vi "Core_Module.vi"(11 "Error_In":errorcluster) -> (4 "Obtained_PSRR_Data":T1, 6 "Last_Read_PSRR (dB)":i32, 8 "Last_Error_Details":T4 caption="Last Error Details", 14 "Colors [4]":T3={"Error?_Color"=[], "Error?_Text"="No_Error"}, 15 "Error_Out":errorcluster)   [LabVIEW 2021]
doc: "Core module perform most of the execution of the application."
uses:
  <vilib>/regexp/Match Regular Expression.xnode
  Controls/Last_Error_Details.ctl
  Controls/BI_Error_Con.ctl
  Controls/Obtained_PSRR_Data.ctl
  Controls/Obtained_PSRR_Data_Operation.ctl
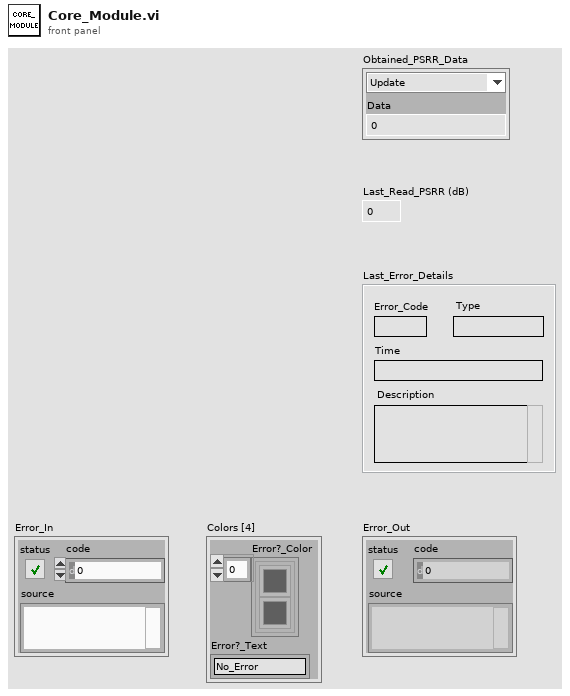
[diagram p1: front panel]
types:
  T1 = typedef "Obtained_PSRR_Data.ctl" = cluster{"Data":i32, "Obtained_PSRR_Data_Operation":T2}
  T2 = typedef "Obtained_PSRR_Data_Operation.ctl" = enum16{"Update", "Dont_Update", "Clear"}
  T3 = typedef "BI_Error_Con.ctl" = cluster{"Error?_Color":cluster{u32, u32}[], "Error?_Text":string}
  T4 = typedef "Last_Error_Details.ctl" = cluster{"Error_Code":string, "Type":string, "Time":string, "Description":string}
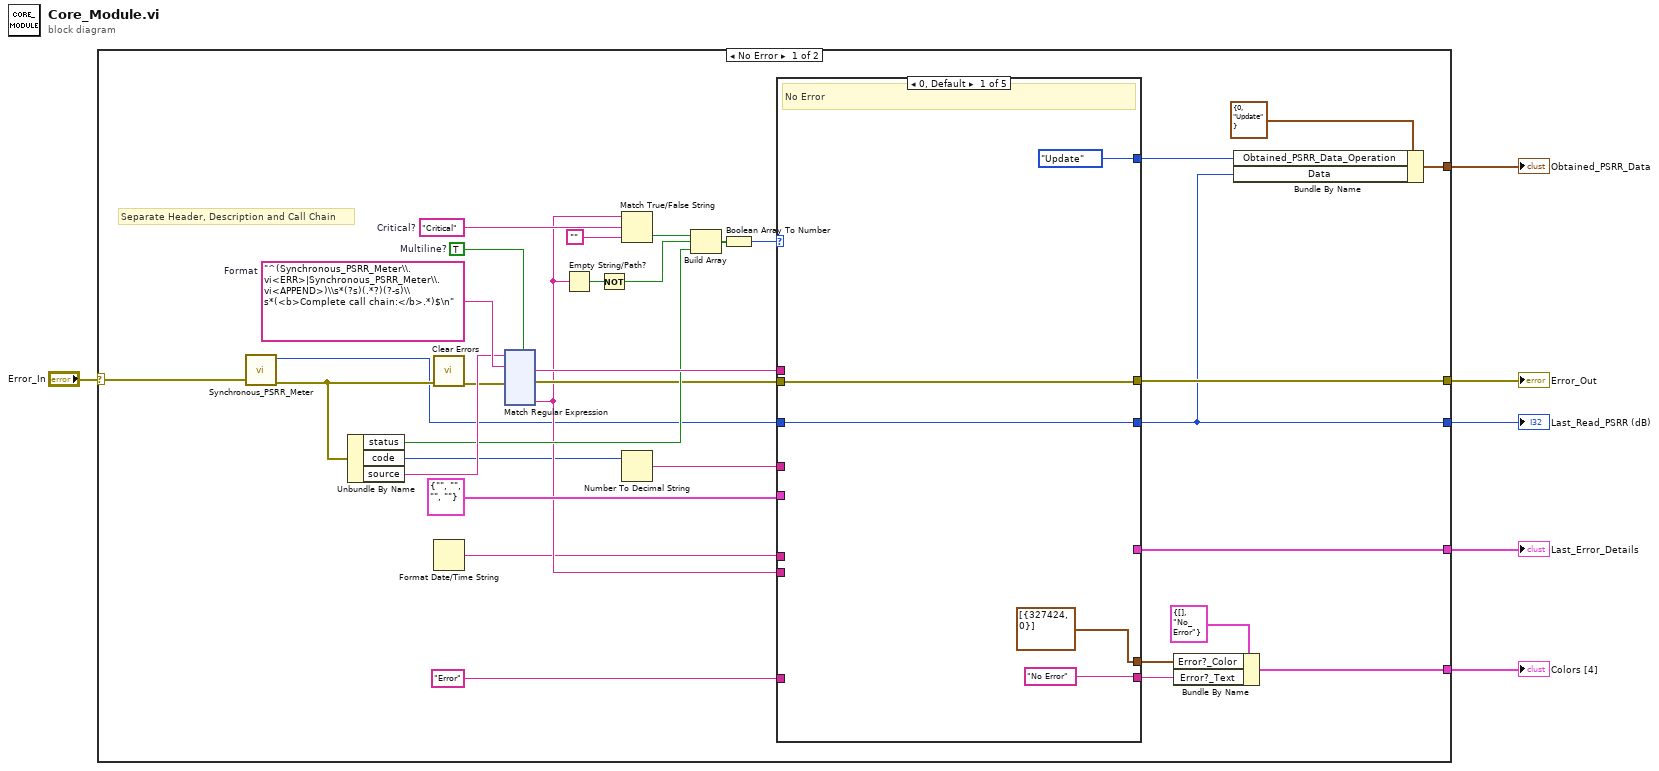
[diagram p0: block diagram]
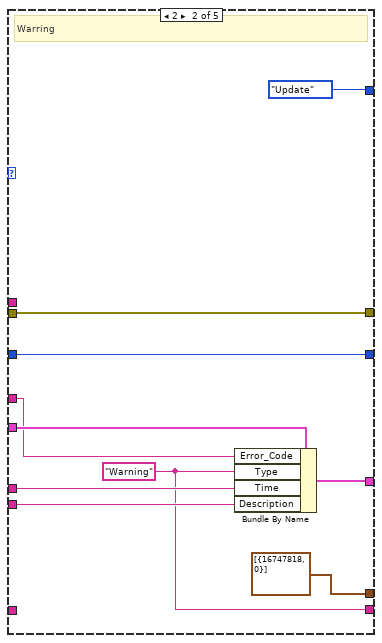
[diagram p2: hidden frame]
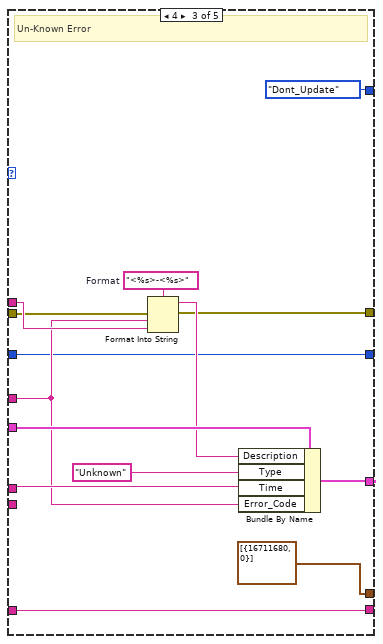
[diagram p3: hidden frame]
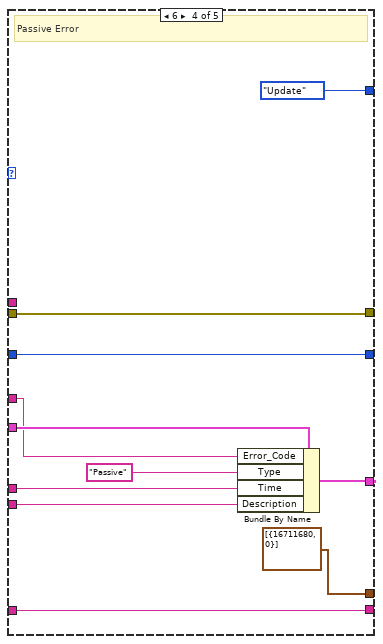
[diagram p4: hidden frame]
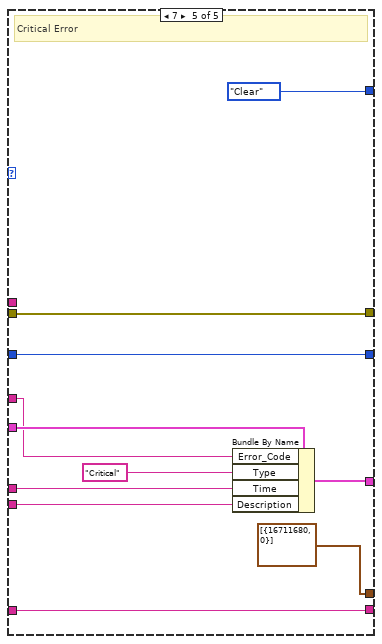
[diagram p5: hidden frame]
diagram:
  n1 = case shown="No Error" "Error_In" {
    selector: "Error_In" -> [w7 w211]
    tunnel: [w26 w211] -> w2
    tunnel: [w12 _] -> w5
    tunnel: [w15 _] -> w6
    tunnel: [w14 _] -> w4
    tunnel: [w19 _] -> w3
    frame No Error {
      w36 = "Critical"  # Critical?
      w38 = TRUE  # Multiline?
      w39 = "^(Synchronous_PSRR_Meter\\.vi<ERR>|Synchronous_PSRR_Meter\\.vi<APPEND>)\\s*(?s)(.*?)(?-s)\\s*(<b>Complete call chain:</b>.*)$\n"  # Format
      # "Separate Header, Description and Call Chain"
      n2 = call "Synchronous_PSRR_Meter.vi"("error in"=w7) -> ("error out"=w9:errorcluster, "PSRR (dB)"=w8:i32)  [unwired: 9 in]
      n3 = Unbundle By Name(w9) -> ("status"=w29:bool, "code"=w22:i32, "source"=w33:string)
      n4 = call <vilib>:"Clear Errors.vi"("error in (no error)"=w9) -> ("error out"=w20:errorcluster)  [unwired: 5 in, 1 out]
      n5 = Format Date/Time String() -> (date/time string=w10:string)  [unwired: 3 in]
      n6 = xnode "Match Regular Expression"("input string"=w33, "regular expression"=w39, "error in"=w20, "multiline? (F)"=w38) -> ("after match"=w37:string, "error out"=w25:errorcluster, "submatch 2"=w24:string)  [unwired: 2 in, 4 out]
      n7 = Empty String/Path?(string/path=w24) -> (empty?=w34:bool)
      n8 = Not(x=w34) -> (.not. x?=w27:bool)
      n9 = Match True/False String(2:"" ("false string"), 3:w36, 4:w24) -> (0:w28:bool)  [unwired: 1 out]
      n10 = Number To Decimal String(number=w22) -> (decimal integer string=w21:string)  [unwired: 1 in]
      n11 = Build Array(w28, w27, w29) -> (w32:bool[])
      n12 = Boolean Array To Number(Boolean array=w32) -> (number=w31:u32)
      n13 = case shown="0, Default" w31 {
        tunnel: w8 -> [w164 w170 w180 w190 w207]
        tunnel: w24 -> [_ w173 _ w197 w208]
        tunnel: w37 -> [_ _ w185 _ _]
        tunnel: T4 {"Error_Code"="", "Type"="", "Time"="", "Description"=""} ("Last_Error_Details") -> [_ w174 w187 w199 w210]
        tunnel: [w163 w169 w178 w194 w204] -> w26
        tunnel: [w164 w170 w180 w190 w207] -> w12
        tunnel: w25 -> [w163 w169 w183 w194 w204]
        tunnel: w10 -> [_ w172 w182 w198 w206]
        tunnel: "Error" ("BoolText.Text") -> [_ _ w176 w191 w201]
        tunnel: w21 -> [_ w171 w181 w195 w205]
        tunnel: [_ w168 w179 w193 w203] -> w19
        tunnel: ["No Error" ("BoolText.Text") w167 w176 w191 w201] -> w18
        tunnel: [cluster{u32, u32}[] [{327424, 0}] ("Colors [4]") cluster{u32, u32}[] [{16747818, 0}] ("Colors [4]") cluster{u32, u32}[] [{16711680, 0}] ("Colors [4]") cluster{u32, u32}[] [{16711680, 0}] ("Colors [4]") cluster{u32, u32}[] [{16711680, 0}] ("Colors [4]")] -> w16
        tunnel: [Obtained_PSRR_Data_Operation."Update" Obtained_PSRR_Data_Operation."Update" Obtained_PSRR_Data_Operation."Dont_Update" Obtained_PSRR_Data_Operation."Update" Obtained_PSRR_Data_Operation."Clear"] -> w11
        frame 0, Default {
          # "No Error"
        }
        frame 2 {
          w167 = "Warning"
          # "Warring"
          n14 = Bundle By Name(cluster=w174, "Error_Code"=w171, "Type"=w167, "Time"=w172, "Description"=w173) -> (w168:T4)
        }
        frame 4 {
          w186 = "<%s>-<%s>"  # Format
          # "Un-Known Error"
          n15 = Format Into String(format string=w186, error in=w183, w181, w185) -> (resulting string=w184:string, error out=w178:errorcluster)  [unwired: 1 in]
          n16 = Bundle By Name(cluster=w187, "Description"=w184, "Type"="Unknown", "Time"=w182, "Error_Code"=w181) -> (w179:T4)
        }
        frame 6 {
          # "Passive Error"
          n17 = Bundle By Name(cluster=w199, "Error_Code"=w195, "Type"="Passive", "Time"=w198, "Description"=w197) -> (w193:T4)
        }
        frame 7 {
          # "Critical Error"
          n18 = Bundle By Name(cluster=w210, "Error_Code"=w205, "Type"="Critical", "Time"=w206, "Description"=w208) -> (w203:T4)
        }
      }
      n19 = Bundle By Name(cluster=T3 {"Error?_Color"=[], "Error?_Text"="No_Error"} ("Colors [4]"), "Error?_Color"=w16, "Error?_Text"=w18) -> (w15:T3)
      n20 = Bundle By Name(cluster=T1 {"Data"=0, "Obtained_PSRR_Data_Operation"=enum."Update"} ("Obtained_PSRR_Data"), "Obtained_PSRR_Data_Operation"=w11, "Data"=w12) -> (w14:T1)
    }
    frame Error {
    }
  }
  "Error_Out" <- w2
  "Last_Read_PSRR (dB)" <- w5
  "Last_Error_Details" <- w3
  "Colors [4]" <- w6
  "Obtained_PSRR_Data" <- w4
